vi "analyseImage.vi"(8 "error in (no error)":errorcluster, 10 "Array":T1(array[cluster]), 11 "AbsorptionDS in":refnum<class "Absorption2.lvclass">) -> (0 "error out":errorcluster, 3 "AbsorptionDS out":refnum<class "Absorption2.lvclass">)   [LabVIEW 2011, in "Tools.lvlib" / "Imaging.lvlib" / "Absorption2.lvclass"]
uses:
  Absorption2.lvclass
  Filing/FileNeologist/FileNeologist.lvclass
  ImageAnalyser.lvclass
  Filing/FileSystem/FileSystem.lvclass
  Imaging.lvlib
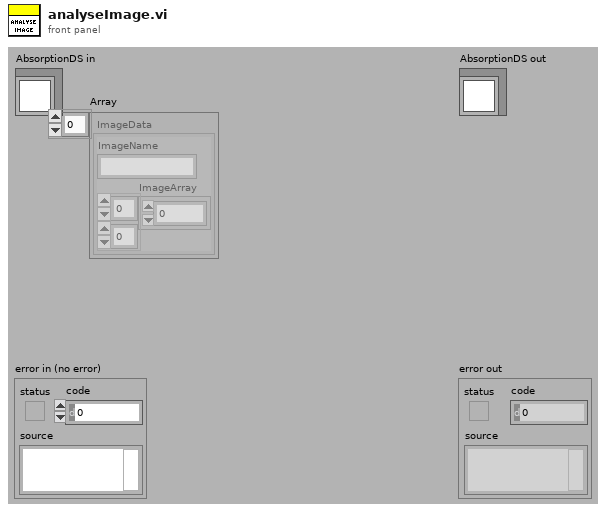
[diagram p1: front panel]
types:
  T1 = cluster{"ImageName":string, "ImageArray":sgl[][]}[]
  T2 = cluster{"Name":string, "Results":dbl[], "AnalysisType":string}
  T3 = cluster{"Left":i32, "Top":i32, "Right":i32, "Bottom":i32}
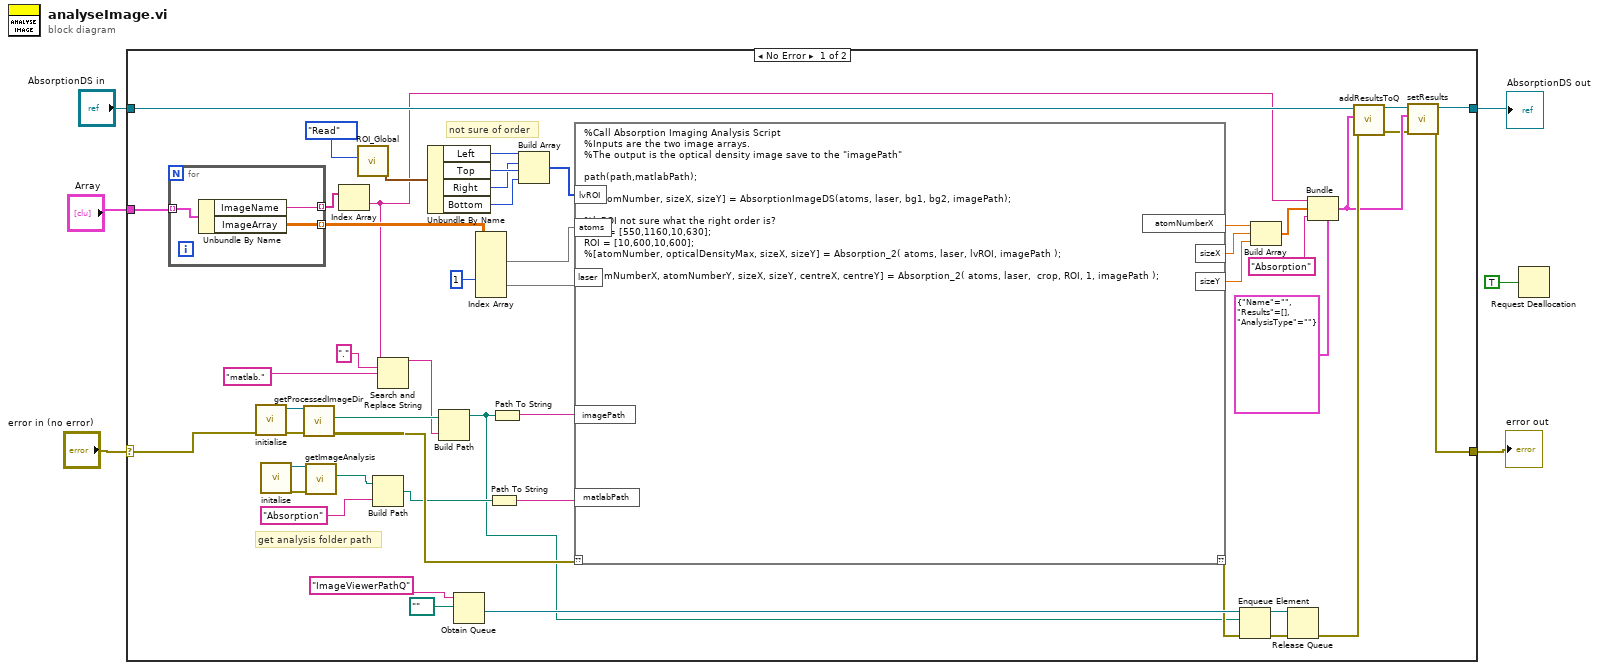
[diagram p0: block diagram]
diagram:
  n1 = case shown="No Error" "error in (no error)" {
    selector: "error in (no error)" -> [w33 w60]
    tunnel: [w21 w60] -> w4
    tunnel: [w24 w59] -> w3
    tunnel: "AbsorptionDS in" -> [w55 w59]
    tunnel: "Array" -> [w54 _]
    frame No Error {
      # "not sure of order"
      # "get analysis folder path"
      n2 = for {
        tunnel: w54 -> [w58] mode=indexing
        tunnel: [w57] -> w53 mode=indexing
        tunnel: [w56] -> w50 mode=indexing
        n3 = Unbundle By Name(w58) -> ("ImageName"=w56:string, "ImageArray"=w57:sgl[][])
      }
      n4 = call "initialise.vi"("error in (no error)"=w33) -> ("error out"=w48:errorcluster, "FileNeologist out"=w49:refnum<class "FileNeologist.lvclass">)  [unwired: 9 in]
      n5 = call "initalise.vi"() -> ("error out"=w29:errorcluster, "FileSystem out"=w30:refnum<class "FileSystem.lvclass">)  [unwired: 10 in]
      n6 = call-dynamic "getProcessedImageDir.vi"("error in (no error)"=w48, "FileNeologist in"=w49) -> ("error out"=w32:errorcluster, "Path"=w47:path)  [unwired: 7 in, 1 out]
      n7 = call "getImageAnalysis.vi"("error in (no error)"=w29, "FileSystem in"=w30) -> ("ImageAnalysis"=w28:path)  [unwired: 7 in, 2 out]
      n8 = Index Array(array=w50) -> (element=w12:string)  [unwired: 1 in]
      n9 = call "ROI_Global.vi"("Action"=enum16{"Write", "Read"}."Read") -> ("ROI"=w18:T3)  [unwired: 10 in]
      n10 = Build Path(base path=w28, name or relative path="Absorption") -> (appended path=w26:path)
      n11 = Search and Replace String(input string=w12, search string=".", replace string="matlab.") -> (result string=w9:string)  [unwired: 5 in, 3 out]
      n12 = Unbundle By Name(w18) -> ("Left"=w17:i32, "Top"=w16:i32, "Right"=w15:i32, "Bottom"=w14:i32)
      n13 = Build Path(base path=w47, name or relative path=w9) -> (appended path=w7:path)
      n14 = Obtain Queue(name (unnamed)="ImageViewerPathQ", element data type=path "") -> (queue out=w44:refnum<queue>)  [unwired: 3 in, 2 out]
      n15 = Index Array(array=w53, index (dim 0) #2=1) -> (element #1=w20:sgl[][], element #2=w51:sgl[][])  [unwired: 5 in]
      n16 = Path To String(path=w26) -> (string=w31:string)
      n17 = Path To String(path=w7) -> (string=w8:string)
      n18 = Build Array(w17, w15, w16, w14) -> (w13:i32[])
      n19 = script code="%Call Absorption Imaging Analysis Script \n%Inputs are the two image arrays.\n%The output is the optical density image save to the \"imagePath\"\n\npath(path,matlabPath);\n\n%[atomNumber, sizeX, sizeY] = AbsorptionImageDS(atoms, laser, bg1, bg2, imagePath);\n\n%lvROI not sure what the right order is? \ncrop = [550,1160,10,630];\nROI = [10,600,10,600];\n%[atomNumber, opticalDensityMax, sizeX, sizeY] = Absorption_2( atoms, laser, lvROI, imagePath );\n\n[atomNumberX, atomNumberY, sizeX, sizeY, centreX, centreY] = Absorption_2( atoms, laser,  crop, ROI, 1, imagePath );"("??"=w32, "laser"=w51, "atoms"=w20, "imagePath"=w8, "matlabPath"=w31, "lvROI"=w13) -> ("??"=w38:errorcluster, "atomNumberX"=w41:dbl, "sizeX"=w40:dbl, "sizeY"=w39:dbl)
      n20 = Enqueue Element(queue=w44, element=w7, error in (no error)=w38) -> (queue out=w43:refnum<queue>, error out=w42:errorcluster)  [unwired: 1 in, 1 out]
      n21 = Build Array(w41, w40, w39) -> (w36:dbl[])
      n22 = Release Queue(queue=w43, error in (no error)=w42) -> (error out=w37:errorcluster)  [unwired: 1 in, 2 out]
      n23 = Bundle(cluster=T2 {"Name"="", "Results"=[], "AnalysisType"=""} ("output cluster"), "Name"=w12, "Results"=w36, "AnalysisType"="Absorption") -> (w23:T2)
      n24 = call "addResultsToQ.vi"("error in (no error)"=w37, "Results"=w23, "ImageAnalyser in"=w55) -> ("error out"=w22:errorcluster, "ImageAnalyser out"=w25:refnum<class "Absorption2.lvclass">)  [unwired: 7 in]
      n25 = call "setResults.vi"("error in (no error)"=w22, "results"=w23, "ImageAnalyser in"=w25) -> ("error out"=w21:errorcluster, "ImageAnalyser out"=w24:refnum<class "Absorption2.lvclass">)  [unwired: 7 in]
    }
    frame Error {
    }
  }
  "error out" <- w4
  "AbsorptionDS out" <- w3
  n26 = Request Deallocation(TRUE ("flag")) -> ()
